vi "getOffsetToTAI.vi"(10 "Epoch Time":i64=2272060800, 11 "Epoch":refnum<class "Epoch.lvclass">) -> (2 "Offset to TAI":i64)   [LabVIEW 2018, in "Epoch.lvclass"]
uses:
  Epoch.lvclass
  leapSeconds LUT.vi
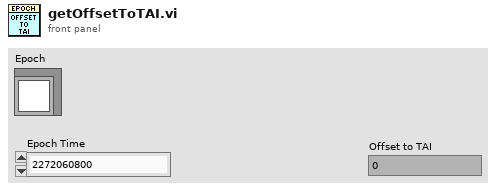
[diagram p1: front panel]
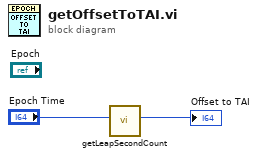
[diagram p0: block diagram]
diagram:
  n1 = call "getLeapSecondCount.vi"("UTC Epoch Time"="Epoch Time") -> ("Leap Seconds"=→"Offset to TAI":i64)  [unwired: 10 in]
